vi "CTRE_ServoBlock_Wait.vi"(10 "Timeout":dbl) -> ()   [LabVIEW 2016]
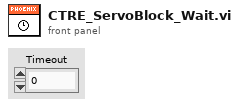
[diagram p1: front panel]
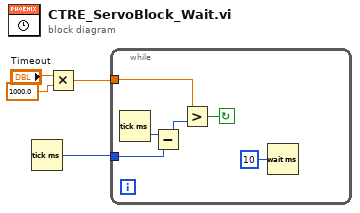
[diagram p0: block diagram]
diagram:
  n1 = Tick Count (ms)() -> (millisecond timer value=w4:u32)
  n2 = Multiply(x="Timeout", y=1000.0) -> (x*y=w1:dbl)
  n3 = while {
    tunnel: w4 -> [w9]
    tunnel: w1 -> [w7]
    stop <- w6 continue-if-true
    n4 = Tick Count (ms)() -> (millisecond timer value=w10:u32)
    n5 = Subtract(x=w10, y=w9) -> (x-y=w8:u32)
    n6 = Greater?(x=w7, y=w8) -> (0:w6:bool)
    n7 = Wait (ms)(milliseconds to wait=u32 10) -> ()  [unwired: 1 out]
  }
